vi "setup_sample.vi"(8 "Flush Volume (mL)":dbl=1.0 min=0.0 max=2.5 step=0.1, 9 "Syringe Flushes":i32=3, 10 "Sample Port":u16(ring)=2 items=["B"=2, "C"=3, "D"=4, "E"=5, "F"=6, "G"=7, "H"=8], 11 "session bundle in":T1={"relay session out"={"VISA resource out"="COM12", "error out"={"status"=FALSE, "code"=0, "source"=""}}, "kloehn session out"={"VISA resource out"="COM12", "error out"={"status"=FALSE, "code"=0, "source"=""}}, "LiCor session out"={"VISA resource out"="COM12", "error out"={"status"=FALSE, "code"=0, "source"=""}}}) -> (0 "kloehn error out":errorcluster, 1 "relay error out":errorcluster, 2 "sample_id":string, 3 "session bundle out":T1={"relay session out"={"VISA resource out"="COM12", "error out"={"status"=FALSE, "code"=0, "source"=""}}, "kloehn session out"={"VISA resource out"="COM12", "error out"={"status"=FALSE, "code"=0, "source"=""}}, "LiCor session out"={"VISA resource out"="COM12", "error out"={"status"=FALSE, "code"=0, "source"=""}}}, 4 "LiCor error out":errorcluster)   [LabVIEW 2010]
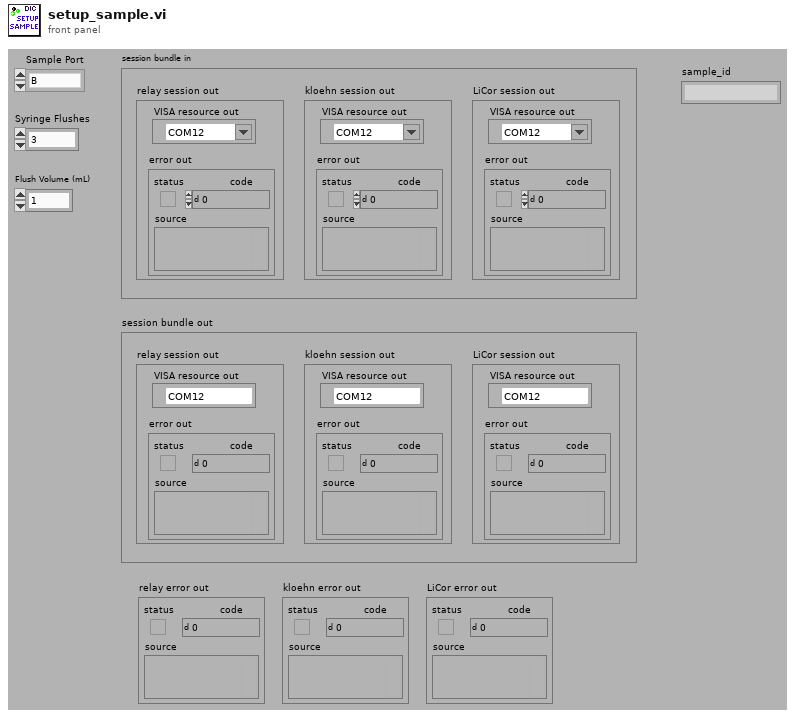
[diagram p1: front panel]
types:
  T1 = cluster{"relay session out":cluster{"VISA resource out":refnum<visa-resource-name>, "error out":errorcluster}, "kloehn session out":cluster{"VISA resource out":refnum<visa-resource-name>, "error out":errorcluster}, "LiCor session out":cluster{"VISA resource out":refnum<visa-resource-name>, "error out":errorcluster}}
  T2 = cluster{"VISA resource out":refnum<visa-resource-name>, "error out":errorcluster}
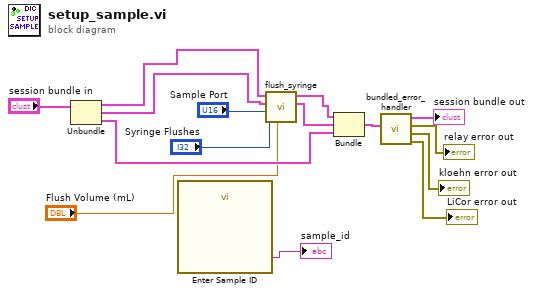
[diagram p0: block diagram]
diagram:
  n1 = Unbundle("session bundle in") -> ("relay session out"=w1:T2, "kloehn session out"=w12:T2, "LiCor session out"=w10:T2)
  n2 = call "Enter Sample ID"() -> ("sample id"=→"sample_id":string)  [unwired: 17 in, 2 out]
  n3 = call "flush_syringe.vi"("Flush Volume (mL)"="Flush Volume (mL)", "Syringe Flushes"="Syringe Flushes", "Sample Port"="Sample Port", "kloehn session in"=w12, "relay session in"=w1) -> ("kloehn session out"=w8:T2, "relay session out"=w9:T2)  [unwired: 5 in]
  n4 = Bundle("relay session out"=w9, "kloehn session out"=w8, "LiCor session out"=w10) -> (w7:T1)  [unwired: 1 in]
  n5 = call "bundled_error_handler.vi"("session bundle in"=w7) -> ("LiCor error out"=→"LiCor error out":errorcluster, "kloehn error out"=→"kloehn error out":errorcluster, "relay error out"=→"relay error out":errorcluster, "session bundle out"=→"session bundle out":T1)  [unwired: 7 in]
